vi "Add Settings.vi"(0 "Configuration Session in":refnum<class "Configuration Session.lvclass">, 1 "id":string, 7 "values":T1, 11 "error in (no error)":errorcluster) -> (4 "Configuration Session out":refnum<class "Configuration Session.lvclass">, 6 "plugin exists?":bool, 15 "error out":errorcluster)   [LabVIEW 2017, in "DSF Core.lvlib" / "Configuration Session.lvclass"]
uses:
  Configuration Session.lvclass
  Public/Controls/DSF Settings Info.ctl
  Configuration Session.lvclass/Configuration Session.ctl
  Controls/DSF File Format/Internal DSF Settings with ID.ctl
  Controls/DSF File Format/Internal DSF Settings Info.ctl
  DSF Core.lvlib
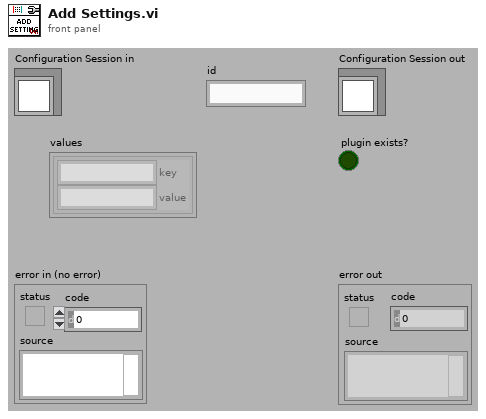
[diagram p1: front panel]
types:
  T1 = typedef "DSF Core.lvlib/DSF Settings Info.ctl" = cluster{"key":string, "value":string}[]
  T2 = typedef "DSF Core.lvlib/Configuration Session.lvclass/Internal DSF Settings with ID.ctl" = cluster{"id":string, "values":T3}
  T3 = typedef "DSF Core.lvlib/Configuration Session.lvclass/Internal DSF Settings Info.ctl" = cluster{"key":string, "value":string}[]
  T4 = typedef "DSF Core.lvlib/Configuration Session.lvclass/DSF Config Data Ref.ctl" = refnum<data-value>
  T5 = typedef "DSF Core.lvlib/Configuration Session.lvclass/DSF Config Data.ctl" = cluster{"dsf configuration":T6, "path":path, "dirty":bool}
  T6 = typedef "DSF Core.lvlib/Configuration Session.lvclass/Internal DSF Configuration.ctl" = cluster{"dsfversion":T7, "version":T7, "plugins":T8[], "groups":T11[], "transfers":T13[], "channels":T15[], "settings":T2[]}
  T7 = typedef "DSF Core.lvlib/DSF Version Info.ctl" = cluster{"major":u32, "minor":u32, "fix":u32, "build":string}
  T8 = typedef "DSF Core.lvlib/Configuration Session.lvclass/Internal DSF Plugin with ID.ctl" = cluster{"id":string, "values":T9}
  T9 = typedef "DSF Core.lvlib/Configuration Session.lvclass/Internal DSF Plugin Info.ctl" = cluster{"type":string, "timing":T10, "group ids":string[], "settings id":string, "thread count":i32}
  T10 = typedef "DSF Core.lvlib/DSF Timing Info.ctl" = cluster{"priority":u64, "decimation":u64, "offset":u64}
  T11 = typedef "DSF Core.lvlib/Configuration Session.lvclass/Internal DSF Group with ID.ctl" = cluster{"id":string, "values":T12}
  T12 = typedef "DSF Core.lvlib/Configuration Session.lvclass/Internal DSF Group Info.ctl" = cluster{"direction":i32, "timing":T10, "transfer ids":string[], "settings id":string}
  T13 = typedef "DSF Core.lvlib/Configuration Session.lvclass/Internal DSF Transfer with ID.ctl" = cluster{"id":string, "values":T14}
  T14 = typedef "DSF Core.lvlib/Configuration Session.lvclass/Internal DSF Transfer Info.ctl" = cluster{"byte order":i32, "channel ids":string[], "settings id":string}
  T15 = typedef "DSF Core.lvlib/Configuration Session.lvclass/Internal DSF Channel with ID.ctl" = cluster{"id":string, "values":T16}
  T16 = typedef "DSF Core.lvlib/Configuration Session.lvclass/Internal DSF Channel Info.ctl" = cluster{"count":u64, "buffer offset":u64, "data type":i32, "settings id":string}
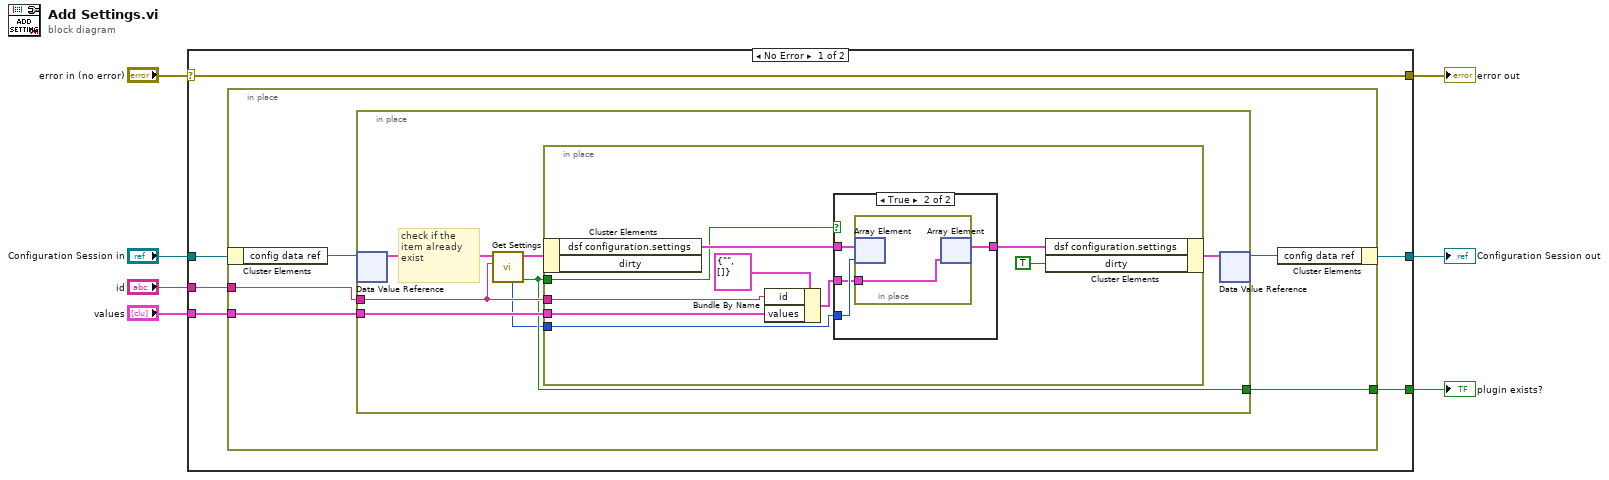
[diagram p0: block diagram]
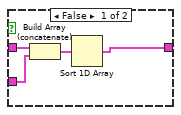
[diagram p2: hidden frame]
diagram:
  n1 = case shown="No Error" "error in (no error)" {
    selector: "error in (no error)" -> [w13 w45]
    tunnel: [w13 w45] -> w6
    tunnel: [w8 w44] -> w1
    tunnel: "Configuration Session in" -> [w9 w44]
    tunnel: "id" -> [w12 _]
    tunnel: "values" -> [w11 _]
    tunnel: [w10 _] -> w3
    frame No Error {
      n2 = in-place {
        in-place-border: w12 -> [w18]
        in-place-border: w11 -> [w17]
        in-place-border: [w16] -> w10
        n3 = in-place-cluster #1(w9) -> ("config data ref"=w15:T4)
        n4 = in-place {
          in-place-border: w18 -> [w25]
          in-place-border: w17 -> [w23]
          in-place-border: [w22] -> w16
          # "check if the item already exist"
          n5 = in-place-dvr #2(w15) -> (w19:T5)  [unwired: 1 out]
          n6 = call "Get Settings.vi"("id"=w25, "DSF Configuration in"=w19) -> ("exists?"=w22:bool, "DSF Configuration out"=w24:T5, "index"=w21:i32)  [unwired: 6 in, 1 out]
          n7 = in-place {
            in-place-border: w25 -> [w33]
            in-place-border: w23 -> [w31]
            in-place-border: w22 -> [w30]
            in-place-border: w21 -> [w29]
            n8 = in-place-cluster #3(w24) -> ("dsf configuration.settings"=w34:T2[])  [unwired: 1 out]
            n9 = Bundle By Name(cluster=T2 {"id"="", "values"=[]} ("settings"), "id"=w33, "values"=w31) -> (w27:T2)
            n10 = case shown="True" w30 {
              tunnel: w34 -> [w38 w42]
              tunnel: [w37 w39] -> w32
              tunnel: w29 -> [_ w41]
              tunnel: w27 -> [w35 w40]
              frame False {
                n11 = Build Array (concatenate)(w38, w35) -> (w36:T2[])
                n12 = Sort 1D Array(array=w36) -> (sorted array=w37:T2[])
              }
              frame True {
                n13 = in-place {
                  in-place-border: w40 -> [w43]
                  n14 = in-place-array #4(w42, w41) -> ()  [unwired: 1 out]
                  n15 = in-place-array #4(w43) -> (w39:T2[])  [unwired: 1 out]
                }
              }
            }
            n16 = in-place-cluster #3("dsf configuration.settings"=w32, "dirty"=TRUE) -> (w20:T5)
          }
          n17 = in-place-dvr #2(w20) -> (w14:T4)  [unwired: 1 out]
        }
        n18 = in-place-cluster #1("config data ref"=w14) -> (w8:refnum<class "Configuration Session.lvclass">)
      }
    }
    frame Error {
    }
  }
  "error out" <- w6
  "plugin exists?" <- w3
  "Configuration Session out" <- w1
